vi "Temperature Controlle2r.vi"() -> ()   [LabVIEW 2010]
panel:
  out "Kelvin Reading":dbl min=0.0 max=1645.0 step=1e-05 format="%^.5e"
  in  "Setpoint (0.0000)":dbl min=-273.0 max=300000.0 step=0.0001 format="%.4f"
  in  "Heater Range (0: Off)":u16(ring) items=["Off", "Low (0.5W)", "Med (5W)", "High (50W)"]
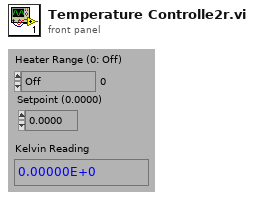
[diagram p1: front panel]
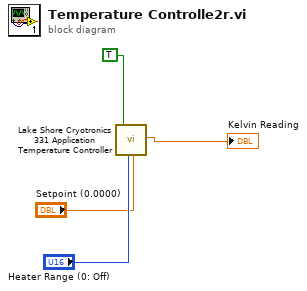
[diagram p0: block diagram]
diagram:
  n1 = call "Lake Shore Cryotronics 331 Application Temperature Controller.vi"("Configure (False)"=TRUE, "Heater Range (0: Off)"="Heater Range (0: Off)", "Setpoint (0.0000)"="Setpoint (0.0000)") -> ("Kelvin Reading"=→"Kelvin Reading":dbl)  [unwired: 13 in, 3 out]
